vi "CE14. Read_kvar(subVI).vi"(8 "error in (no error)":errorcluster, 9 "milliseconds to wait(100)":u32=100, 11 "VISA resource name":refnum<visa-resource-name>) -> (0 "error out":errorcluster, 1 "data out":T1, 2 "read buffer":string, 3 "VISA resource name out":refnum<visa-resource-name>)   [LabVIEW 2018, in "CE14_eMIC.lvlib"]
uses:
  CE14_eMIC.lvlib
  type defs/CE14.data.ctl
  <vilib>/Instr/_visa.llb/VISA Flush IO Buffer Mask.ctl
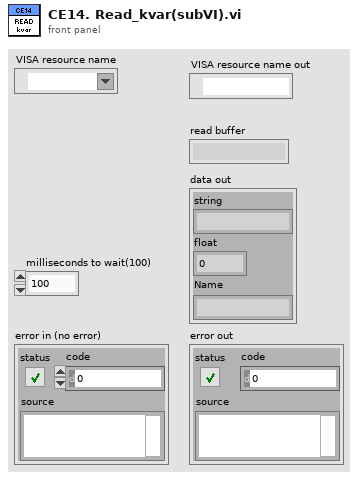
[diagram p1: front panel]
types:
  T1 = typedef "CE14_eMIC.lvlib/CE14.data.ctl" = cluster{"string":string, "float":dbl, "Name":string}
  T2 = typedef "VISA Flush IO Buffer Mask.ctl" = u16
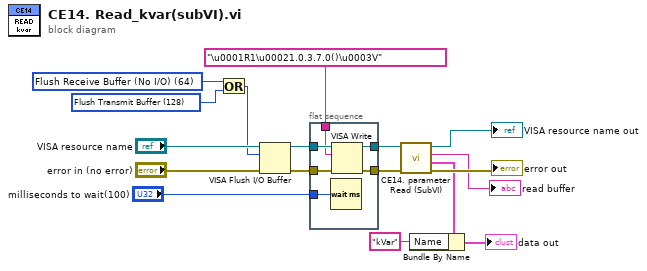
[diagram p0: block diagram]
diagram:
  w5 = T2 128 items=["Flush Receive Buffer"=16, "Write Transmit Buffer to Device"=32, "Flush Receive Buffer (No I/O)"=64, "Flush Transmit Buffer"=128] ("Mask")
  w6 = T2 64 items=["Flush Receive Buffer"=16, "Write Transmit Buffer to Device"=32, "Flush Receive Buffer (No I/O)"=64, "Flush Transmit Buffer"=128] ("Mask")
  n1 = Or(x=w6, y=w5) -> (x .or. y?=w4:T2)
  n2 = VISA Flush I/O Buffer(VISA resource name="VISA resource name", mask (16)=w4, error in (no error)="error in (no error)") -> (VISA resource name out=w8:refnum<visa-resource-name>, error out=w9:errorcluster)
  n3 = flat-sequence {
    tunnel: w8 -> [w23]
    tunnel: w9 -> [w22]
    tunnel: [w21] -> w16
    tunnel: [w20] -> w17
    tunnel: "\u0001R1\u00021.0.3.7.0()\u0003V" -> [w19]
    tunnel: "milliseconds to wait(100)" -> [w18]
    frame #0 {
      n4 = Wait (ms)(milliseconds to wait=w18) -> ()  [unwired: 1 out]
      n5 = VISA Write(VISA resource name=w23, write buffer=w19, error in (no error)=w22) -> (VISA resource name out=w20:refnum<visa-resource-name>, error out=w21:errorcluster)  [unwired: 1 out]
    }
  }
  n6 = call "CE14. parameter Read (SubVI).vi"("error in (no error)"=w16, "VISA Refnum in"=w17) -> ("error out"=→"error out":errorcluster, "dataout"=w3:T1, "read buffer"=→"read buffer":string, "VISA Refnum out"=→"VISA resource name out":refnum<visa-resource-name>)  [unwired: 5 in, 1 out]
  n7 = Bundle By Name(cluster=w3, "Name"="kVar") -> (→"data out":T1)
